vi "Create Circle.vi"(6 "Color Box":u32(colorbox)=5878015, 8 "error in (no error)":errorcluster, 9 "Radius":i32=3, 10 "Position":cluster{"Left":i32, "Top":i32}={"Left"=32, "Top"=32}, 11 "Circle in":refnum<class "Circle.lvclass">) -> (0 "error out":errorcluster, 3 "Circle out":refnum<class "Circle.lvclass">)   [LabVIEW 2015, in "Circle.lvclass"]
uses:
  Circle.lvclass
  <vilib>/LIEF/Forms/Shape/Shape.lvclass/Shape.ctl
  <vilib>/LIEF/Forms/Shape/Write Color.vi
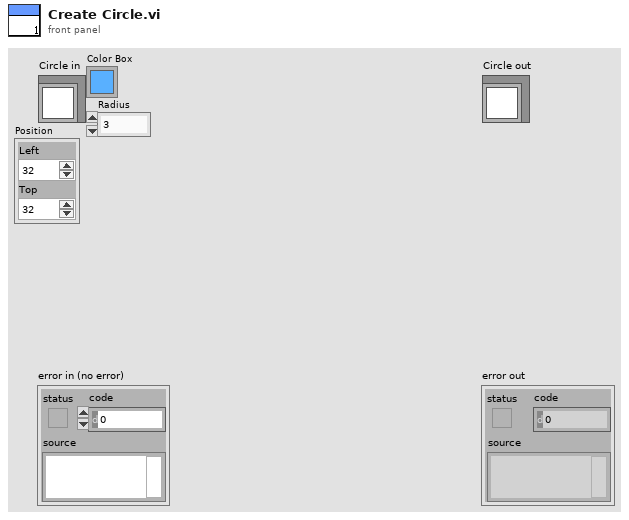
[diagram p1: front panel]
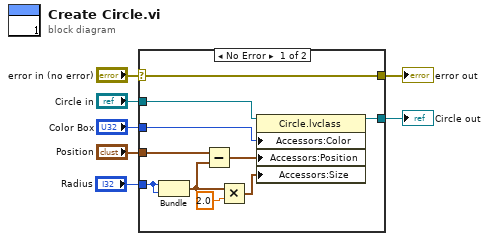
[diagram p0: block diagram]
diagram:
  n1 = case shown="No Error" "error in (no error)" {
    selector: "error in (no error)" -> [w17 w19]
    tunnel: [w17 w19] -> w6
    tunnel: [w13 w18] -> w4
    tunnel: "Circle in" -> [w14 w18]
    tunnel: "Position" -> [w12 _]
    tunnel: "Radius" -> [w11 _]
    tunnel: "Color Box" -> [w9 _]
    frame No Error {
      n2 = Bundle("Radius"=w11, "Radius"=w11) -> (w8:cluster{"Radius":i32, "Radius":i32})  [unwired: 1 in]
      n3 = Subtract(x=w12, y=w8) -> (x-y=w16:cluster{i32, i32})
      n4 = Multiply(x=w8, y=2.0 ("x")) -> (x*y=w10:cluster{"Radius":dbl, "Radius":dbl})
      n5 = property class="Circle.lvclass"(reference=w14, "Accessors:Color"=w9, "Accessors:Position"=w16, "Accessors:Size"=w10) -> (reference out=w13:refnum<class "Circle.lvclass">)  [unwired: 1 in, 1 out]
    }
    frame Error {
    }
  }
  "error out" <- w6
  "Circle out" <- w4
